vi "hidSPD Error Handler.vi"(8 "error in (no error)":errorcluster, 10 "hidSPD Viewer State in":T1, 11 "spdDevSessions in":T2[](array[typedef])) -> (0 "error out":errorcluster, 2 "hidSPD Viewer State out":T1, 3 "spdDevSessions out":T2[](array[typedef]))   [LabVIEW 2018, in "hidSPDLibForLabView.lvlib"]
uses:
  hidSPDLibForLabView.lvlib
  hidSPD Controls/hidSPD Device Session.ctl
  hidSPD Controls/hidSPD Viwer State.ctl
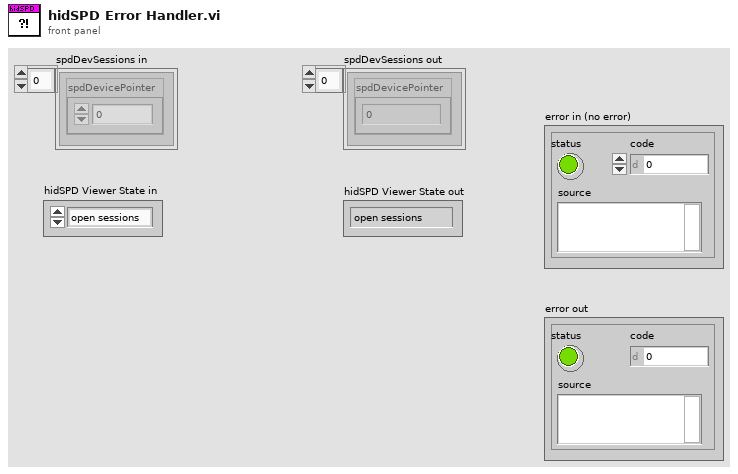
[diagram p1: front panel]
types:
  T1 = typedef "hidSPDLibForLabView.lvlib/hidSPD Viwer State.ctl" = enum16{"open sessions", "close sessions", "read reports"}
  T2 = typedef "hidSPDLibForLabView.lvlib/hidSPD Device Session.ctl" = cluster{"spdDevicePointer":u64}
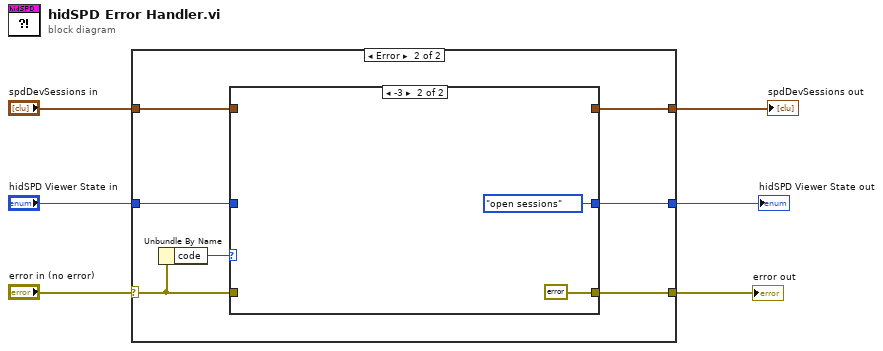
[diagram p0: block diagram]
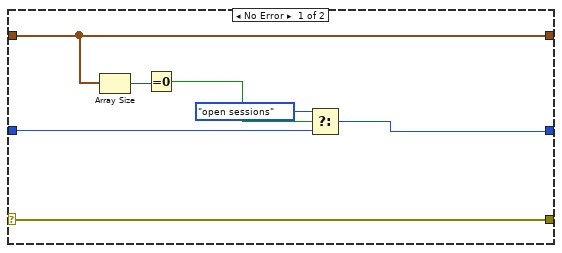
[diagram p2: hidden frame]
diagram:
  n1 = case shown="Error" "error in (no error)" {
    selector: "error in (no error)" -> [w13 w17]
    tunnel: [w13 w16] -> w5
    tunnel: [w12 w14] -> w3
    tunnel: "spdDevSessions in" -> [w12 w15]
    tunnel: "hidSPD Viewer State in" -> [w9 w19]
    tunnel: [w7 w18] -> w1
    frame No Error {
      n2 = Array Size(array=w12) -> (size(s)=w11:i32)
      n3 = Equal To 0?(x=w11) -> (x = 0?=w10:bool)
      n4 = Select(t=hidSPD_Viwer_State."open sessions", s=w10, f=w9) -> (s? t:f=w7:T1)
    }
    frame Error {
      n5 = Unbundle By Name(w17) -> ("code"=w20:i32)
      n6 = case shown="-3" w20 {
        tunnel: w19 -> [w23 _]
        tunnel: [w23 hidSPD_Viwer_State."open sessions" ("hidSPD Viewer State in")] -> w18
        tunnel: [w22 errorcluster {"status"=FALSE, "code"=0, "source"=""} ("error IO")] -> w16
        tunnel: w17 -> [w22 _]
        tunnel: w15 -> [w21 _]
        tunnel: [w21 _] -> w14
        frame 0, Default {
        }
        frame -3 {
        }
      }
    }
  }
  "error out" <- w5
  "spdDevSessions out" <- w3
  "hidSPD Viewer State out" <- w1
